vi "Cluster Array.vi"(8 "Error In":errorcluster) -> (0 "Error Out":errorcluster)   [LabVIEW 2018, in "Tests.lvlib" / "To Msgpack.lvlib"]
uses:
  To Msgpack.lvlib
  <vilib>/addons/_JKI Toolkits/Caraya/classes/Test/Test.lvclass
  src/Toolkit/Toolkit.lvlib
  <vilib>/addons/_JKI Toolkits/Caraya/classes/Assert/Assert.lvclass
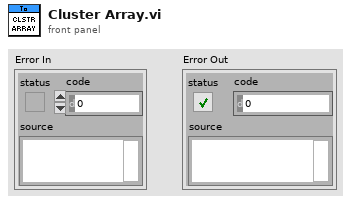
[diagram p1: front panel]
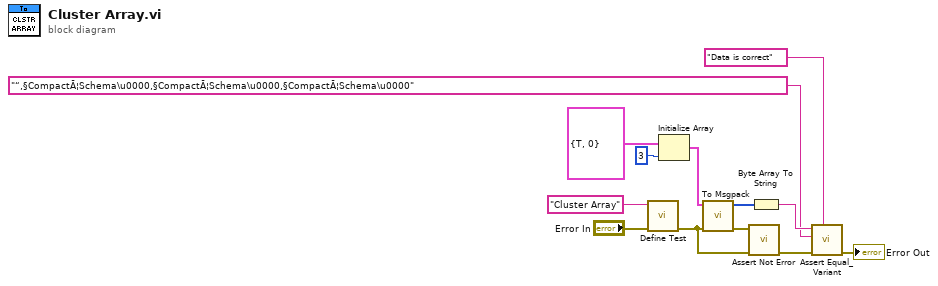
[diagram p0: block diagram]
diagram:
  n1 = call <vilib>:"Define Test.vi"("error in (no error)"="Error In", "Label (VI Title)"="Cluster Array") -> ("error out"=w9:errorcluster)  [unwired: 9 in]
  n2 = Initialize Array(cluster{"Compact":bool, "Schema":i32} {"Compact"=TRUE, "Schema"=0}, 3 ("dimension size")) -> (w1:cluster{"Compact":bool, "Schema":i32}[])
  n3 = call "To Msgpack.vi"("Error In"=w9, "Anything"=w1) -> ("Error Out"=w10:errorcluster, "Msgpack Data"=w7:u8[])  [unwired: 8 in]
  n4 = call <vilib>:"Assert Not Error.vi"("error in (no error)"=w9, "Not Error?"=w10) -> ("error out"=w11:errorcluster)  [unwired: 9 in]
  n5 = Byte Array To String(unsigned byte array=w7) -> (string=w6:string)
  n6 = call <vilib>:"Assert Equal_Variant.vi"("Label"="Data is correct", "error in (no error)"=w11, "Y"="“‚§CompactÃ¦Schema\u0000‚§CompactÃ¦Schema\u0000‚§CompactÃ¦Schema\u0000" ("string"), "X"=w6) -> ("error out"=→"Error Out":errorcluster)  [unwired: 7 in]
